vi "dll.midi_file_get_info.vi"(8 "error in (no error)":errorcluster, 11 "midi file in":refnum<class "midi file.lvclass">) -> (0 "error out":errorcluster, 2 "File Info Cluster":T1, 3 "midi file out":refnum<class "midi file.lvclass">)   [LabVIEW 2020, in "MIDIllan.lvlib" / "midi file.lvclass"]
uses:
  midi file.lvclass
  file info.ctl
  midi file.lvclass/midi file.ctl
  MIDIllan/MIDIllan.lvlib
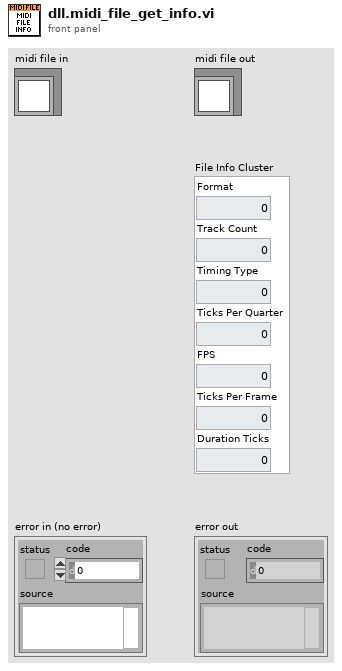
[diagram p1: front panel]
types:
  T1 = typedef "MIDIllan.lvlib/midi file.lvclass/file info.ctl" = cluster{"Format":i32, "Track Count":i32, "Timing Type":i32, "Ticks Per Quarter":i32, "FPS":sgl, "Ticks Per Frame":i32, "Duration Ticks":u32}
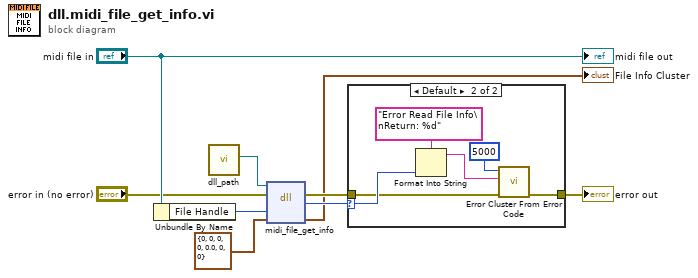
[diagram p0: block diagram]
diagram:
  n1 = Unbundle By Name("midi file in") -> ("File Handle"=w5:i32)
  n2 = call "dll_path.vi"() -> ("dll"=w9:path)  [unwired: 11 in]
  n3 = dll-call lib="C:/code/LabVIEW-MIDI-XPLAT/dist/TomMIDIllan_*.*" fn="midi_file_get_info"(path in=w9, error in="error in (no error)", "File Handle"=w5, "File Info Cluster"=T1 {"Format"=0, "Track Count"=0, "Timing Type"=0, "Ticks Per Quarter"=0, "FPS"=0.0, "Ticks Per Frame"=0, "Duration Ticks"=0} ("File Info")) -> (error out=w8:errorcluster, "Error code"=w7:i32, "File Info Cluster"=→"File Info Cluster":T1)  [unwired: 2 in, 1 out]
  n4 = case shown="Default" w7 {
    selector: w7 -> [_ w13]
    tunnel: w8 -> [w10 w12]
    tunnel: [w10 w11] -> w1
    frame 0.. {
    }
    frame Default {
      n5 = Format Into String(format string="Error Read File Info\nReturn: %d", w13) -> (resulting string=w14:string)  [unwired: 2 in, 1 out]
      n6 = call <vilib>:"Error Cluster From Error Code.vi"("error in (no error)"=w12, "error message (\"\")"=w14, "error code (0)"=5000) -> ("error out"=w11:errorcluster)  [unwired: 6 in]
    }
  }
  "error out" <- w1
  "midi file out" <- "midi file in"
